vi "修改预设波形.vi"(9 "一炮最长运行时间":dbl, 10 "波形点":cluster{"时间点":dbl, "幅值":dbl}, 11 "原预设波形":dbl[][](array[numeric])) -> (2 "修改后波形":dbl[][](array[numeric]))   [LabVIEW 2018]
uses:
  9bcc4e12-daf4-48db-95f4-256412c0a8f5.vi
  <vilib>/Array/Sort 2D Array - Pop Stack.vi
  <vilib>/Array/Sort 2D Array - Push Stack.vi
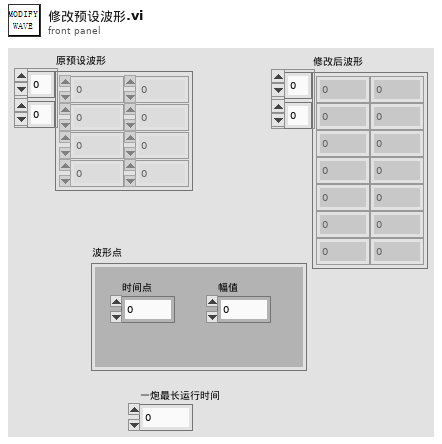
[diagram p1: front panel]
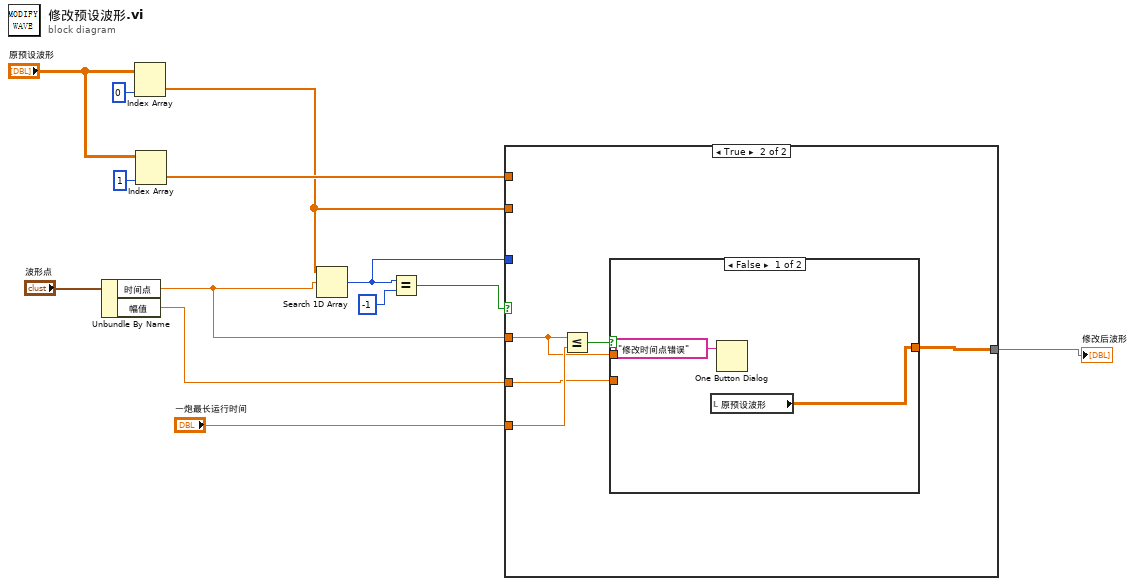
[diagram p0: block diagram]
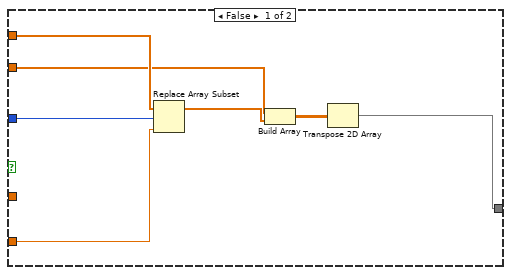
[diagram p2: hidden frame]
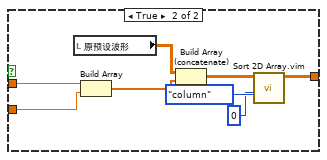
[diagram p3: hidden frame]
diagram:
  n1 = Unbundle By Name("波形点") -> ("时间点"=w9:dbl, "幅值"=w7:dbl)
  n2 = Index Array(array="原预设波形", index (col)=0 ("disabled index (col)")) -> (element=w1:dbl[])  [unwired: 1 in]
  n3 = Index Array(array="原预设波形", index (col)=1 ("disabled index (col)")) -> (element=w3:dbl[])  [unwired: 1 in]
  n4 = Search 1D Array(1D array=w1, element=w9) -> (index of element=w2:i32)  [unwired: 1 in]
  n5 = Equal?(x=w2, y=-1) -> (x = y?=w10:bool)
  n6 = case shown="True" w10 {
    tunnel: w9 -> [_ w23]
    tunnel: "一炮最长运行时间" -> [_ w25]
    tunnel: w7 -> [w18 w22]
    tunnel: [w14 w21] -> w6
    tunnel: w3 -> [w20 _]
    tunnel: w2 -> [w19 _]
    tunnel: w1 -> [w17 _]
    frame False {
      n7 = Replace Array Subset(array=w20, new element=w18, index=w19) -> (w16:dbl[])
      n8 = Build Array(w17, w16) -> (w15:dbl[][])
      n9 = Transpose 2D Array(2D array=w15) -> (transposed array=w14:dbl[][])
    }
    frame True {
      n10 = Less Or Equal?(x=w23, y=w25) -> (x <= y?=w24:bool)
      n11 = case shown="False" w24 {
        tunnel: w23 -> [_ w35]
        tunnel: w22 -> [_ w34]
        tunnel: [w26 w28] -> w21
        frame False {
          n12 = local read "原预设波形"() -> (w26:dbl[][])
          n13 = One Button Dialog(message="修改时间点错误") -> ()  [unwired: 1 in, 1 out]
        }
        frame True {
          n14 = local read "原预设波形"() -> (w33:dbl[][])
          n15 = Build Array(w35, w34) -> (w32:dbl[])
          n16 = Build Array (concatenate)(w33, w32) -> (w31:dbl[][])
          n17 = call "Sort 2D Array.vim"("index"=0, "dimension to index (column)"=enum16{"column", "row"}."column", "2D array"=w31) -> ("sorted 2D array"=w28:dbl[][])  [unwired: 7 in, 1 out]
        }
      }
    }
  }
  "修改后波形" <- w6
